vi "Parse Access String.vi"(11 "String Value":string) -> (3 "reservation access (Read/Write)":i32)   [LabVIEW 2015]
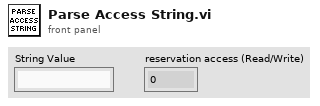
[diagram p1: front panel]
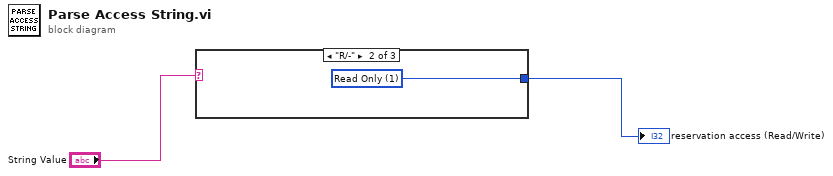
[diagram p0: block diagram]
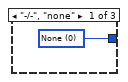
[diagram p2: hidden frame]
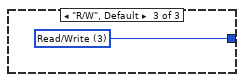
[diagram p3: hidden frame]
diagram:
  n1 = case shown="\"R/-\"" "String Value" {
    tunnel: [w3 w4 w5] -> w1
    frame "-/-", "none" {
      w3 = 0 items=["None"=0, "Read Only"=1, "Read/Write"=3] ("reservation access (Read/Write)")
    }
    frame "R/-" {
      w4 = 1 items=["None"=0, "Read Only"=1, "Read/Write"=3] ("reservation access (Read/Write)")
    }
    frame "R/W", Default {
      w5 = 3 items=["None"=0, "Read Only"=1, "Read/Write"=3] ("reservation access (Read/Write)")
    }
  }
  "reservation access (Read/Write)" <- w1
